vi "Model - Get State.vi"(8 "error in (no error)":errorcluster, 11 "View Model":T2) -> (0 "error out":errorcluster, 1 "Next State":T1, 2 "Current State":T1, 3 "View Model":T2)   [LabVIEW 2017]
doc: "Get actual current and next state values from DVR"
uses:
  Controls/View Model.ctl
  Controls/Shared Model.ctl
  Error/Controls/Error Model.ctl
  Error/Controls/Error Event.ctl
  Error/Controls/Error Type.ctl
  Configuration/Controls/Config DB Model.ctl
  Configuration/Controls/Config DB Command.ctl
  Configuration/Controls/Config DB Record.ctl
  Controller/Controls/Controller Model.ctl
  Controller/Controls/Elevator Location.ctl
  Controller/Controls/Elevator Direction Event.ctl
  Controller/Controls/Elevator Direction.ctl
  Controller/Controls/Elevator CMD Event.ctl
  Controller/Controls/Elevator Commands.ctl
  Controller/Controls/Elevator Overhead.ctl
  Controller/Controls/Elevator State.ctl
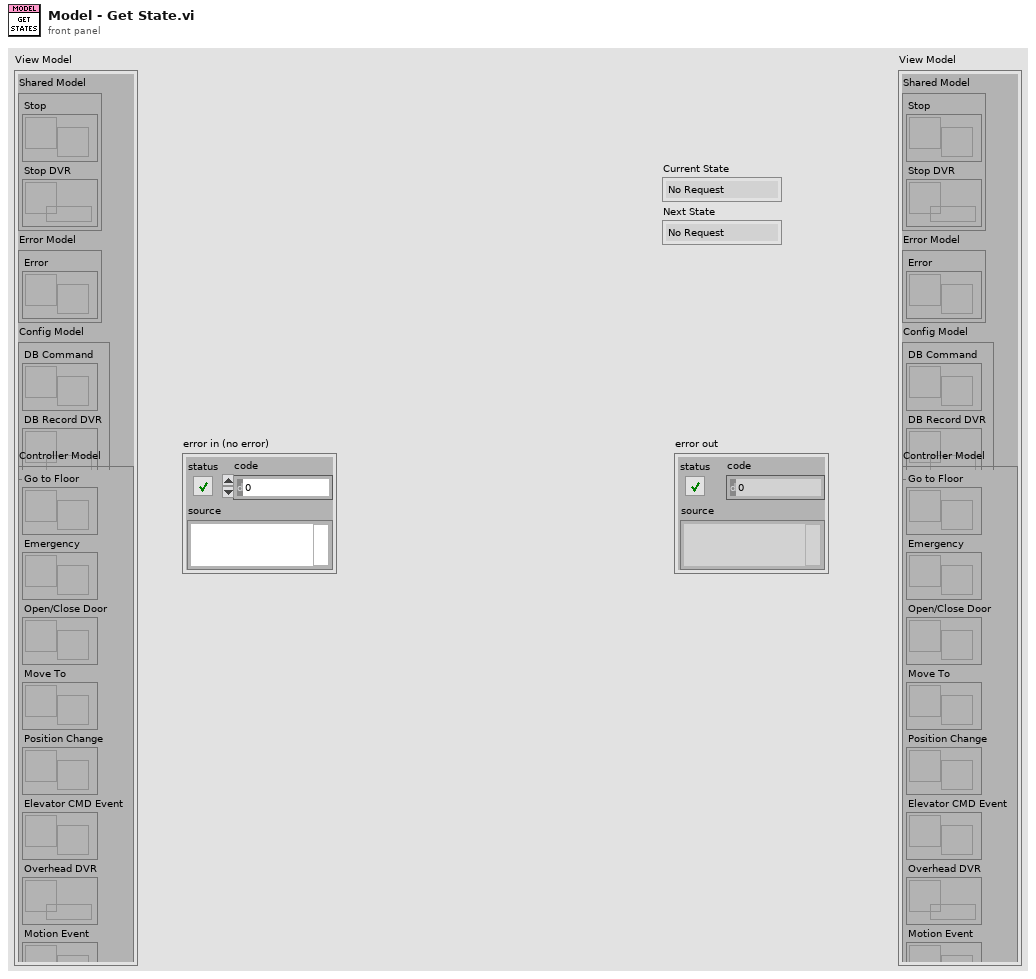
[diagram p1: front panel]
types:
  T1 = typedef "Elevator State.ctl" = enum16{"No Request", "Initial", "Wait for 1st Request", "Start and Move", "Anakysis", "Continue Travel", "Stop at Floor", "Open/Close Door", "Emergency", "Terminate"}
  T2 = typedef "View Model.ctl" = cluster{"Shared Model":T3, "Error Model":T4, "Config Model":T5, "Controller Model":T6}
  T3 = typedef "Shared Model.ctl" = cluster{"Stop":refnum<user-event>, "Stop DVR":refnum<data-value>}
  T4 = typedef "Error Model.ctl" = cluster{"Error":refnum<user-event>}
  T5 = typedef "Config DB Model.ctl" = cluster{"DB Command":refnum<user-event>, "DB Record DVR":refnum<data-value>}
  T6 = typedef "Controller Model.ctl" = cluster{"Go to Floor":refnum<user-event>, "Emergency":refnum<user-event>, "Open/Close Door":refnum<user-event>, "Move To":refnum<user-event>, "Position Change":refnum<user-event>, "Elevator CMD Event":refnum<user-event>, "Overhead DVR":refnum<data-value>, "Motion Event":refnum<user-event>}
  T7 = typedef "Elevator Overhead.ctl" = cluster{"In Motion?":bool, "Direction":bool, "Door Movement":bool, "Current State":T1, "Next State":T1}
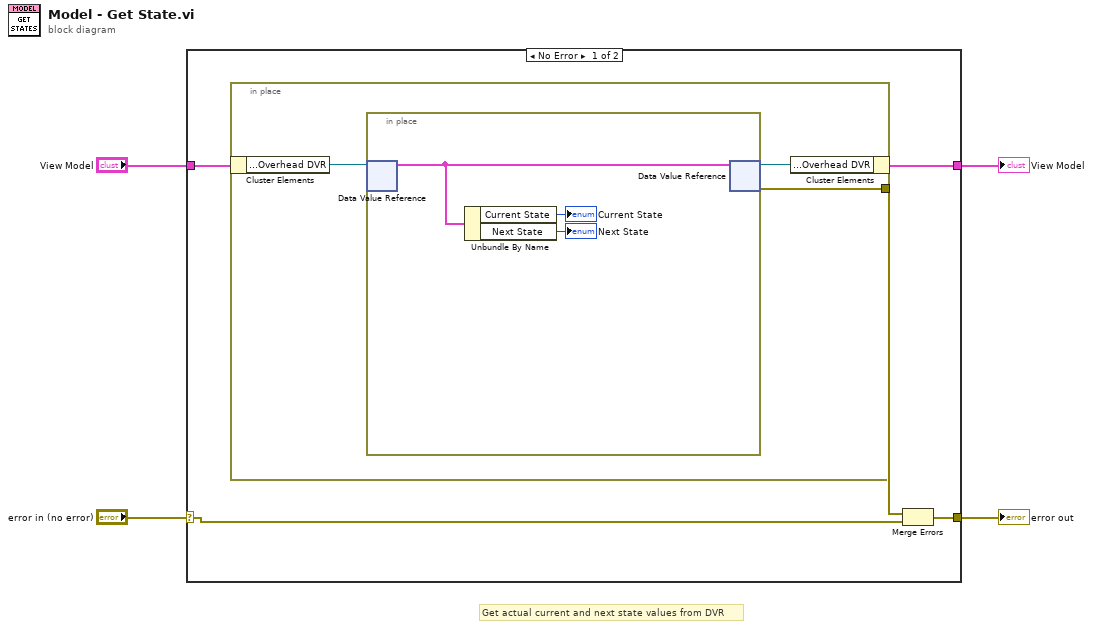
[diagram p0: block diagram]
diagram:
  # "Get actual current and next state values from DVR"
  n1 = case shown="No Error" "error in (no error)" {
    selector: "error in (no error)" -> [w7 w16]
    tunnel: "View Model" -> [w9 w17]
    tunnel: [w8 w17] -> w2
    tunnel: [w6 w16] -> w1
    frame No Error {
      n2 = in-place {
        in-place-border: [w10] -> w5
        n3 = in-place-cluster #1(w9) -> ("Controller Model.Overhead DVR"=w12:refnum<data-value>)
        n4 = in-place {
          n5 = in-place-dvr #2(w12) -> (w15:T7)  [unwired: 1 out]
          n6 = Unbundle By Name(w15) -> ("Current State"=→"Current State":T1, "Next State"=→"Next State":T1)
          n7 = in-place-dvr #2(w15) -> (w11:refnum<data-value>, w10:errorcluster)
        }
        n8 = in-place-cluster #1("Controller Model.Overhead DVR"=w11) -> (w8:T2)
      }
      n9 = Merge Errors(w5, w7) -> (w6:errorcluster)
    }
    frame Error {
    }
  }
  "error out" <- w1
  "View Model" <- w2
